vi "get_name.vi"(8 "error in (no error)":errorcluster, 11 "ClassC in":refnum<class "ClassC.lvclass">) -> (0 "error out":errorcluster, 2 "name":string="ClassC", 3 "ClassC out":refnum<class "ClassC.lvclass">)   [LabVIEW 2010, in "ClassC.lvclass"]
uses:
  ClassC.lvclass
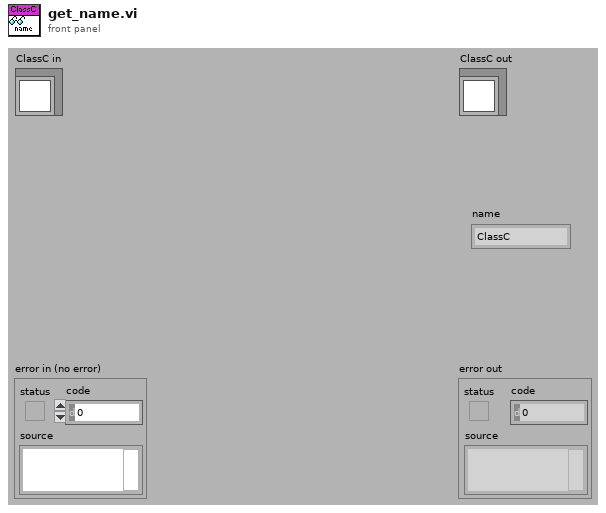
[diagram p1: front panel]
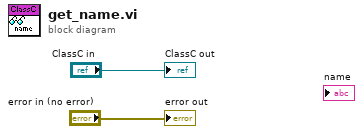
[diagram p0: block diagram]
diagram:
  "error out" <- "error in (no error)"
  "ClassC out" <- "ClassC in"
